vi "Trigger FXP(+,-,18,1)_20221208.vi"(0 "data A":fxp<+/-,18,1>[](array[numeric])=[0.0, 0.0], 1 "reset":bool, 2 "trigger.ready for reference":bool, 5 "data B":fxp<+/-,18,1>[](array[numeric])=[0.0, 0.0], 7 "input valid":bool, 9 "trigger.level Hi":T1, 11 "trigger.level Lo":T1, 12 "trigger.combination type":T5=enum."A", 13 "rearm delay":u16=2) -> (4 "timestamps":T3, 6 "trigger.out":T4, 8 "overflow":bool)   [LabVIEW 2021]
uses:
  FPGA Interface Typedefinitions/Trigger Combination Type.ctl
  <instrlib>/_niInstr/Types/v1/Shared/Public/Input Triggers.ctl
  <instrlib>/_niInstr/Multirecord Acquisition/Interface/v1/FPGA/Public/Timestamp.ctl
  <instrlib>/_niInstr/Data Trigger/v1/Shared/Public/Level Configuration FXP(+-,18,1).ctl
  <instrlib>/_niInstr/Data Trigger/v1/Shared/Public/Level Configuration Trigger When.ctl
  <instrlib>/_niInstr/Data Trigger/v1/FPGA/Private/Trigger/Level FXP(+-,18,1)xNspc.vi
  <instrlib>/_niInstr/Types/v1/Shared/niInstr Types v1 Shared.lvlib
  <instrlib>/_niInstr/Basic Elements/v1/FPGA/niInstr Basic Elements v1 FPGA.lvlib
  <instrlib>/_niInstr/Data Trigger/v1/FPGA/niInstr Data Trigger v1 FPGA.lvlib
  <instrlib>/_niInstr/Multirecord Acquisition/Interface/v1/FPGA/niInstr Multirecord Acquisition v1 FPGA.lvclass
  Trigger Interpolation/Trigger Interpolation FXP(+,-,18,1)x2spc.vi
  <instrlib>/_niInstr/Basic Elements/v1/FPGA/Private/D Latch U16.vi
  <instrlib>/_niInstr/Data Trigger/v1/Shared/niInstr Data Trigger v1 Shared.lvlib
  FPGA Interface Typedefinitions/FPGA Interface Typedefinitions.lvlib
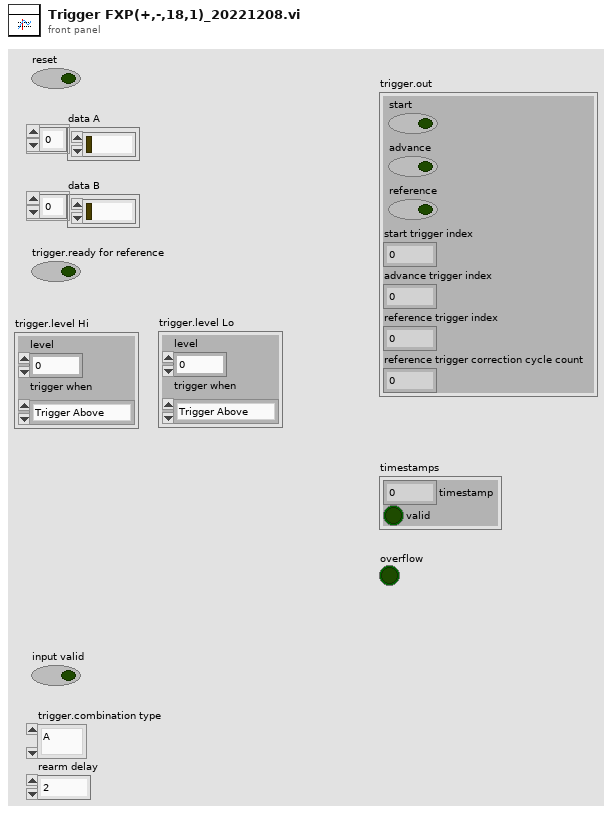
[diagram p1: front panel]
types:
  T1 = typedef "niInstr Data Trigger v1 Shared.lvlib/Level Configuration FXP(+-,18,1).ctl" = cluster{"level":fxp<+/-,18,5>, "trigger when":T2}
  T2 = typedef "niInstr Data Trigger v1 Shared.lvlib/Level Configuration Trigger When.ctl" = enum8{"Trigger Above", "Trigger Below"}
  T3 = typedef "niInstr Multirecord Acquisition v1 FPGA.lvclass/Timestamp.ctl" = cluster{"timestamp":u64, "valid":bool}
  T4 = typedef "niInstr Types v1 Shared.lvlib/Input Triggers.ctl" = cluster{"start":bool, "advance":bool, "reference":bool, "start trigger index":u16, "advance trigger index":u16, "reference trigger index":u16, "reference trigger correction cycle count":u32}
  T5 = typedef "FPGA Interface Typedefinitions.lvlib/Trigger Combination Type.ctl" = enum16{"Immediate", "A", "B", "OR", "AND", "A THEN B", "B THEN A", "High Resolution"}
  T6 = typedef "niInstr Data Trigger v1 Shared.lvlib/Edge Configuration Trigger Slope.ctl" = enum8{"Positive", "Negative"}
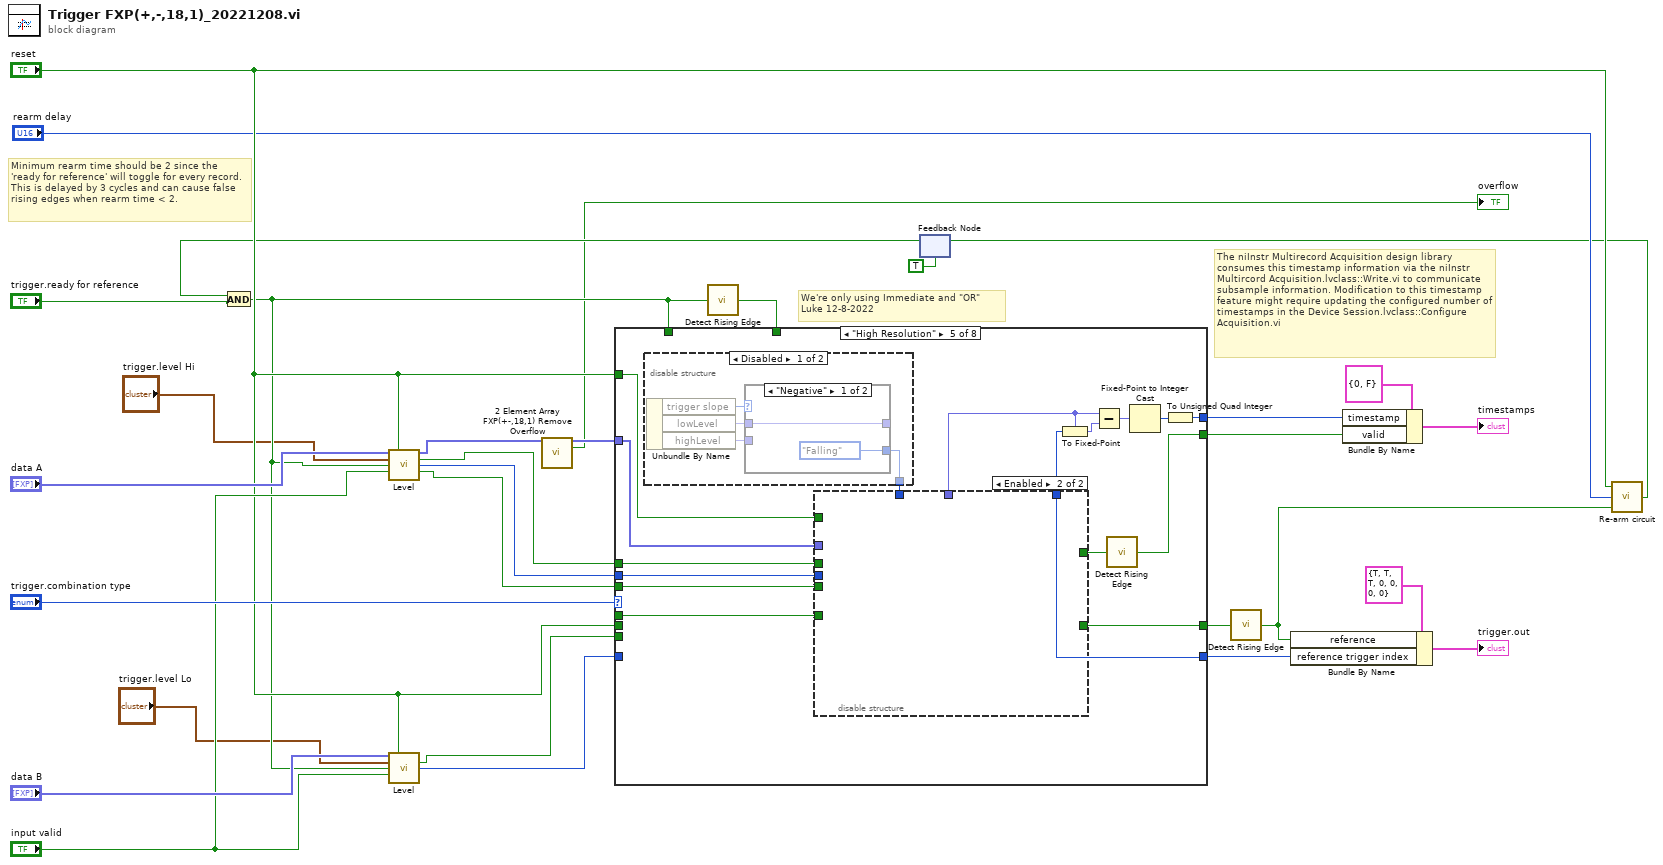
[diagram p0: block diagram]
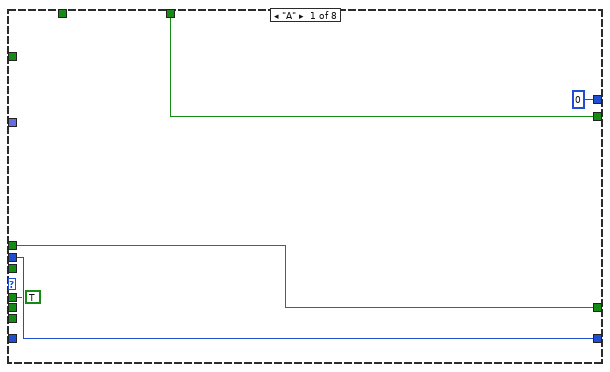
[diagram p2: hidden frame]
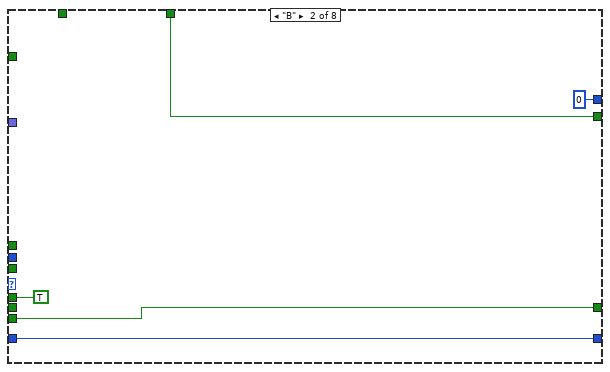
[diagram p3: hidden frame]
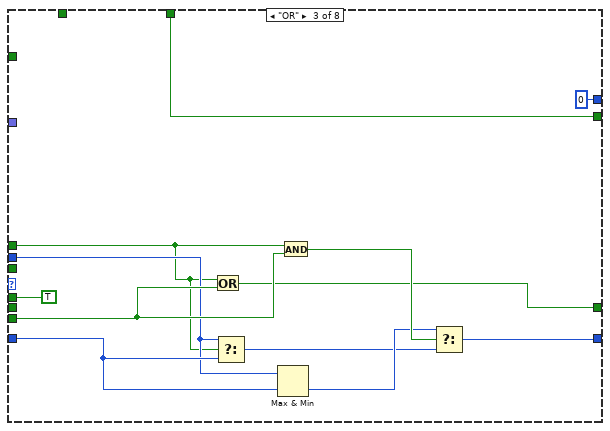
[diagram p4: hidden frame]
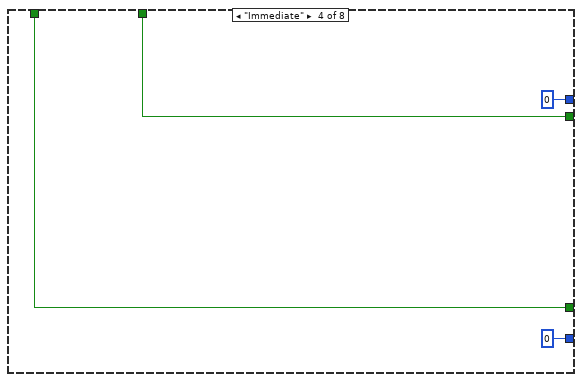
[diagram p5: hidden frame]
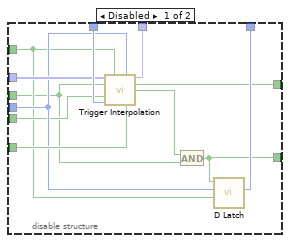
[diagram p6: hidden frame]
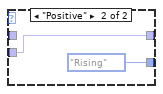
[diagram p7: hidden frame]
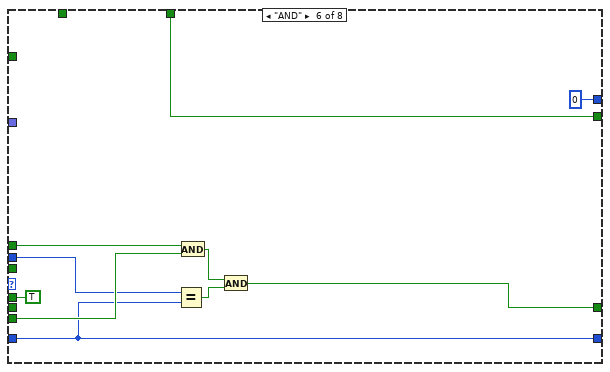
[diagram p9: hidden frame]
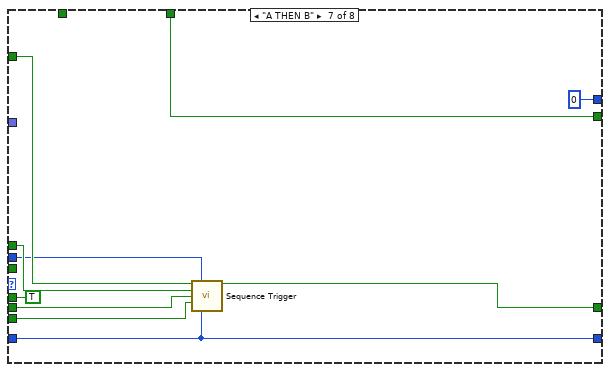
[diagram p10: hidden frame]
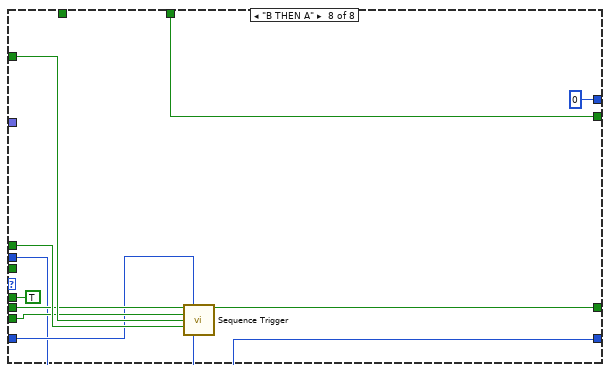
[diagram p11: hidden frame]
diagram:
  # "We're only using Immediate and \"OR\" \nLuke 12-8-2022"
  # "Minimum rearm time should be 2 since the 'ready for reference' will toggle for every record. This is delayed by 3 cycles and can cause false rising edges when rearm time < 2."
  # "The niInstr Multirecord Acquisition design library consumes this timestamp information via the niInstr Multircord Acquisition.lvclass::Write.vi to communicate subsample information. Modification to this timestamp feature might require updating the configured number of timestamps in the Device Session.lvclass::Configure Acquisition.vi"
  n1 = feedback #1(TRUE ("rearm out")) -> (w7:bool)
  n2 = And(x=w7, y="trigger.ready for reference") -> (x .and. y?=w6:bool)
  n3 = call-poly <instrlib>:"Level.vi"("data in"="data A", "reset"="reset", "configuration"="trigger.level Hi", "arm (T)"=w6, "input valid"="input valid") -> ("data out"=w5:fxp<+/-,18,1>[], "trigger"=w24:bool, "trigger index"=w27:u16, "output valid"=w30:bool)  [unwired: 4 in, 3 out]
  n4 = call-poly <instrlib>:"Level.vi"("data in"="data B", "reset"="reset", "configuration"="trigger.level Lo", "arm (T)"=w6, "input valid"="input valid") -> ("trigger"=w25:bool, "trigger index"=w28:u16)  [unwired: 4 in, 5 out]
  n5 = call "2 Element Array FXP(+-,18,1) Remove Overflow.vi"("data in"=w5) -> ("data out"=w4:fxp<+/-,18,1>[], "overflow"=→"overflow":bool)  [unwired: 13 in]
  n6 = call <instrlib>:"Detect Rising Edge.vi"("signal"=w6) -> ("edge detected"=w15:bool)  [unwired: 14 in]
  n7 = case shown="\"High Resolution\"" "trigger.combination type" {
    tunnel: w24 -> [w36 _ w45 _ w59 w103 w112 w121]
    tunnel: w25 -> [_ w41 w47 _ _ w102 w110 w120]
    tunnel: [w36 w41 w44 w55 w58 w98 w109 w123] -> w14
    tunnel: w27 -> [w35 _ w46 _ w64 w101 w105 w114]
    tunnel: w28 -> [_ w40 w48 _ _ w97 w104 w115]
    tunnel: [w35 w40 w43 u16 0 ("trigger index") w66 w97 w104 w114] -> w29
    tunnel: "reset" -> [_ _ _ _ w60 _ w113 w122]
    tunnel: "reset" -> [_ _ _ _ _ _ w111 w119]
    tunnel: w4 -> [_ _ _ _ w65 _ _ _]
    tunnel: w30 -> [_ _ _ _ w63 _ _ _]
    tunnel: [u64 0 ("trigger time") u64 0 ("trigger time") u64 0 ("trigger time") u64 0 ("trigger time") w71 u64 0 ("trigger time") u64 0 ("trigger time") u64 0 ("trigger time")] -> w22
    tunnel: [w32 w37 w52 w54 w61 w94 w106 w116] -> w21
    tunnel: w6 -> [_ _ _ w55 _ _ _ _]
    tunnel: [TRUE ("ready for input") TRUE ("ready for input") TRUE ("ready for input") _ w70 TRUE ("ready for input") TRUE ("ready for input") TRUE ("ready for input")] -> _
    tunnel: w15 -> [w32 w37 w52 w54 _ w94 w106 w116]
    frame "A" {
    }
    frame "B" {
    }
    frame "OR" {
      n8 = Or(x=w45, y=w47) -> (x .or. y?=w44:bool)
      n9 = Select(t=w46, s=w45, f=w48) -> (s? t:f=w49:u16)
      n10 = Max & Min(x=w46, y=w48) -> (min(x,y)=w50:u16)  [unwired: 1 out]
      n11 = And(x=w45, y=w47) -> (x .and. y?=w51:bool)
      n12 = Select(t=w50, s=w51, f=w49) -> (s? t:f=w43:u16)
    }
    frame "Immediate" {
    }
    frame "High Resolution" {
      n13 = disable-structure shown="Disabled" {
        disable-tunnel: [w89 _] -> w73
        frame Disabled {
          n14 = Unbundle By Name() -> ("trigger slope"=w86:T6, "lowLevel"=w88:fxp<+/-,18,1>, "highLevel"=w87:fxp<+/-,18,1>)  [unwired: 1 in]
          n15 = case shown="\"Negative\"" w86 {
            tunnel: [enum16{"Rising", "Falling"}."Falling" ("trigger direction") enum16{"Rising", "Falling"}."Rising" ("trigger direction")] -> w89
            tunnel: [w90 w92] -> _
            tunnel: w88 -> [w90 _]
            tunnel: w87 -> [_ w92]
            frame "Negative" {
            }
            frame "Positive" {
            }
          }
        }
        frame Enabled {
        }
      }
      n16 = disable-structure shown="Enabled" {
        disable-tunnel: w73 -> [w85 _]
        disable-tunnel: [w84 _] -> w70
        disable-tunnel: [w83 _] -> w68
        disable-tunnel: [w82 _] -> w66
        disable-tunnel: w65 -> [w81 _]
        disable-tunnel: w64 -> [w80 _]
        disable-tunnel: w63 -> [w79 _]
        disable-tunnel: [w78 _] -> w62
        disable-tunnel: w60 -> [w77 _]
        disable-tunnel: w59 -> [w76 _]
        disable-tunnel: [w74 _] -> w58
        frame Disabled {
          n17 = call-poly "Trigger Interpolation.vi"("data in"=w81, "reset"=w77, "trigger index"=w80, "trigger"=w76, "data valid"=w79, "trigger direction"=w85) -> ("trigger time"=w83:fxp<+/-,32,5>, "trigger time valid"=w78:bool, "ready for trigger"=w75:bool, "ready for input"=w84:bool)  [unwired: 5 in, 1 out]
          n18 = And(x=w75, y=w76) -> (x .and. y?=w74:bool)
          n19 = call-poly <instrlib>:"D Latch.vi"("r"=w77, "d"=w80, "s"=w74) -> ("q"=w82:u16)  [unwired: 8 in]
        }
        frame Enabled {
        }
      }
      n20 = To Fixed-Point(fixed-point type=w68, number=w66) -> (fixed-point=w69:fxp<+/-,32,5>)
      n21 = Subtract(x=w68, y=w69) -> (x-y=w67:fxp<+/-,33,6>)
      n22 = call <instrlib>:"Detect Rising Edge.vi"("signal"=w62) -> ("edge detected"=w61:bool)  [unwired: 14 in]
      n23 = Fixed-Point to Integer Cast(1:w67) -> (0:w72:i64)
      n24 = To Unsigned Quad Integer(1:w72) -> (0:w71:u64)
    }
    frame "AND" {
      n25 = Equal?(x=w101, y=w97) -> (x = y?=w99:bool)
      n26 = And(x=w103, y=w102) -> (x .and. y?=w100:bool)
      n27 = And(x=w100, y=w99) -> (x .and. y?=w98:bool)
    }
    frame "A THEN B" {
      n28 = call "Sequence Trigger.vi"("reset A"=w113, "trigger index A"=w105, "A"=w112, "reset B"=w111, "B"=w110, "trigger index B"=w104) -> ("trigger"=w109:bool)  [unwired: 9 in]
    }
    frame "B THEN A" {
      n29 = call "Sequence Trigger.vi"("reset A"=w119, "trigger index A"=w115, "A"=w120, "reset B"=w122, "B"=w121, "trigger index B"=w114) -> ("trigger"=w123:bool)  [unwired: 9 in]
    }
  }
  n30 = call <instrlib>:"Detect Rising Edge.vi"("signal"=w14) -> ("edge detected"=w13:bool)  [unwired: 14 in]
  n31 = Bundle By Name(cluster=T4 {"start"=TRUE, "advance"=TRUE, "reference"=TRUE, "start trigger index"=0, "advance trigger index"=0, "reference trigger index"=0, "reference trigger correction cycle count"=0} ("triggers in"), "reference"=w13, "reference trigger index"=w29) -> (→"trigger.out":T4)
  n32 = Bundle By Name(cluster=T3 {"timestamp"=0, "valid"=FALSE} ("timestamp"), "timestamp"=w22, "valid"=w21) -> (→"timestamps":T3)
  n33 = call "Re-arm circuit.vi"("trigger"=w13, "delay"="rearm delay", "reset"="reset") -> ("rearm out"=w10:bool)
  n34 = feedback-in #1(w10) -> ()
